vi "Bin to TDMS.vi"() -> ()   [LabVIEW 2016]
uses:
  resonant_ultrasound/maglab ultrasound -- arkady/file -- scan filename action.ctl
panel:
  out "Date/times":string[](array[string])
  in  "group name in (Untitled)":string="p"
  in  "Frequency scale":dbl=1000.0
  out "Output files":path[](array[path])
  in  "Columns":string[](array[string])=["Frequency", "Signal X", "Signal Y"]
  out "Error Out":errorcluster
  in  "Error In":errorcluster
  in  "Folder Path":path
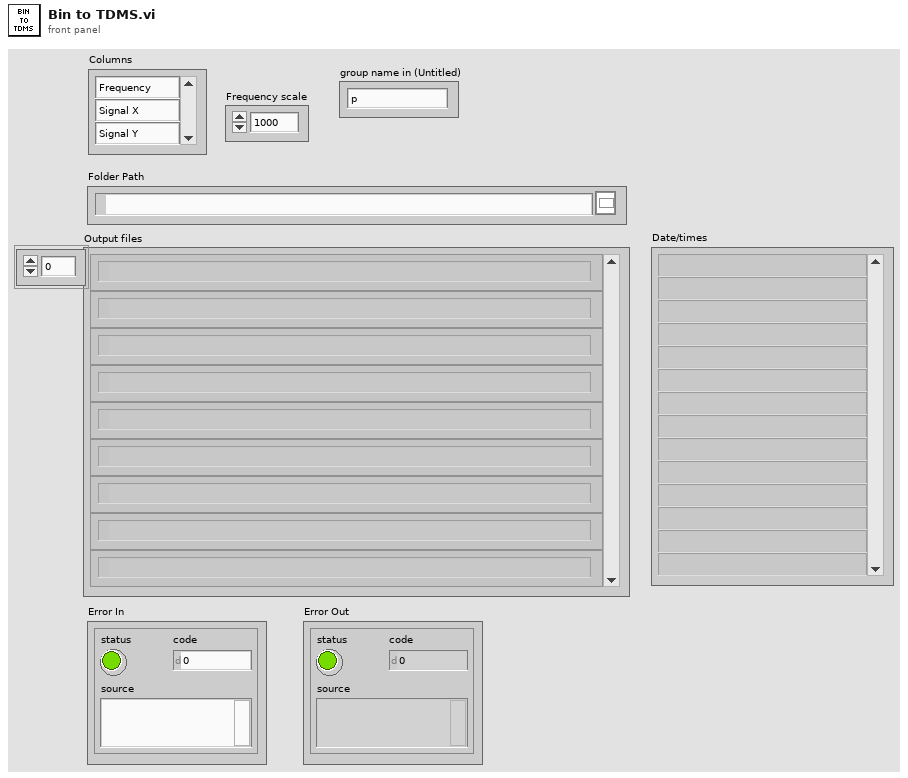
[diagram p1: front panel]
types:
  T1 = typedef "file -- scan filename action.ctl" = enum16{"prefix base name", "datestring regexp", "parse datestring", "datestring", "filename regexp", "parse filename", "datestring regexp (no brackets)", "suffix base name"}
  T2 = enum16{"open", "open or create", "create or replace", "create", "open (read-only)"}
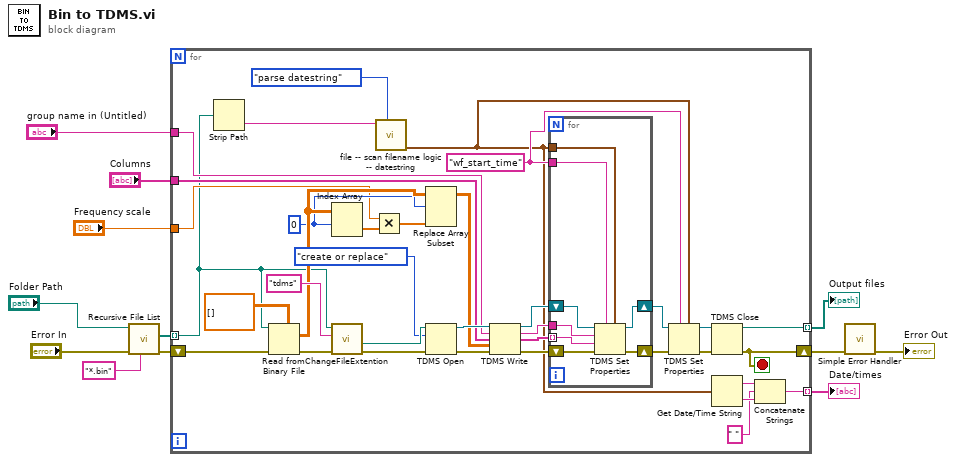
[diagram p0: block diagram]
diagram:
  n1 = call <vilib>:"Recursive File List.vi"("pattern"="*.bin", "error in (no error)"="Error In", "Folder Path"="Folder Path") -> ("error out"=w9:errorcluster, "All Files in Dir"=w4:path[])  [unwired: 4 in, 3 out]
  n2 = for {
    tunnel: w4 -> [w29] mode=indexing
    shift-right: [w41] -> w7
    shift-left: w9 -> [w43]
    tunnel: [w42] -> w8 mode=indexing
    tunnel: "Columns" -> [w40]
    tunnel: "Frequency scale" -> [w31]
    tunnel: "group name in (Untitled)" -> [w30]
    tunnel: [w20] -> w1 mode=indexing
    stop <- w41 stop-if-true
    w14 = "wf_start_time"
    w34 = 0 ("index")
    n3 = Strip Path(path=w29) -> (name=w24:string)  [unwired: 1 out]
    n4 = Read from Binary File(5:dbl[][] [], 8:w43, 11:w29) -> (0:w38:errorcluster, 2:w36:dbl[][])  [unwired: 3 in, 2 out]
    n5 = Index Array(array=w36, index (row)=w34) -> (element=w33:dbl[])  [unwired: 1 in]
    n6 = call "ChangeFileExtention.vi"("Error In"=w38, "New extension"="tdms" ("New Extention"), "File Path"=w29) -> ("Error Out"=w37:errorcluster, "Path with new extension"=w44:path)  [unwired: 3 in, 4 out]
    n7 = Multiply(x=w31, y=w33) -> (x*y=w32:dbl[])
    n8 = call "file -- scan filename logic -- datestring.vi"("scan filename action"=file_--_scan_filename_action."parse datestring", "date/time string IN"=w24) -> ("time stamp OUT"=w13:timestamp)  [unwired: 6 in, 3 out]
    n9 = Replace Array Subset(array=w36, new element=w32, index (row)=w34) -> (w35:dbl[][])  [unwired: 1 in]
    n10 = TDMS Open(8:w37, 10:T2."create or replace" ("operation (0:open)"), 11:w44) -> (0:w46:errorcluster, 3:w45:refnum<k34>)  [unwired: 4 in]
    n11 = TDMS Write(0:w45, 5:w30, 7:w40, 9:w35, 11:w46) -> (4:w28:refnum<k34>, 6:w26:string, 8:w25:string[], 15:w27:errorcluster)  [unwired: 1 in]
    n12 = for {
      tunnel: w14 -> [w56]
      tunnel: w13 -> [w53]
      tunnel: w26 -> [w52]
      tunnel: w25 -> [w51] mode=indexing
      shift-right: [w50] -> w18
      shift-left: w27 -> [w54]
      shift-right: [w49] -> w16
      shift-left: w28 -> [w55]
      n13 = TDMS Set Properties(5:w53, 7:w56, 8:w54, 9:w51, 10:w52, 11:w55) -> (0:w50:errorcluster, 3:w49:refnum<k34>)  [unwired: 2 out]
    }
    n14 = TDMS Set Properties(5:w13, 7:w14, 8:w18, 11:w16) -> (0:w17:errorcluster, 3:w15:refnum<k34>)  [unwired: 2 in, 2 out]
    n15 = TDMS Close(8:w17, 11:w15) -> (0:w41:errorcluster, 3:w42:path)
    n16 = Get Date/Time String(seconds (now)=w13) -> (date string=w21:string, time string=w22:string)  [unwired: 2 in]
    n17 = Concatenate Strings(w21, " " ("string"), w22) -> (w20:string)
  }
  "Output files" <- w8
  "Date/times" <- w1
  n18 = call <vilib>:"Simple Error Handler.vi"("error in (no error)"=w7) -> ("error out"=→"Error Out":errorcluster)  [unwired: 4 in, 4 out]
